vi "r4.vi"   [LabVIEW 2019]
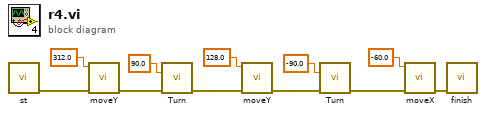
[diagram p0: block diagram]
diagram:
  n1 = call "st.vi"() -> ("Error/Flow Out"=w11:errorcluster)  [unwired: 11 in]
  n2 = call "moveY.vi"("error in (no error)"=w11, "Y"=312.0) -> ("error out"=w9:errorcluster)  [unwired: 9 in]
  n3 = call "Turn.vi"("¨¤«×"=90.0, "error in (no error)"=w9) -> ("error out"=w6:errorcluster)  [unwired: 13 in]
  n4 = call "moveY.vi"("error in (no error)"=w6, "Y"=128.0) -> ("error out"=w4:errorcluster)  [unwired: 9 in]
  n5 = call "Turn.vi"("¨¤«×"=-90.0, "error in (no error)"=w4) -> ("error out"=w3:errorcluster)  [unwired: 13 in]
  n6 = call "moveX.vi"("error in (no error)"=w3, "X"=-60.0) -> ("error out"=w1:errorcluster)  [unwired: 9 in]
  n7 = call "finish.vi"("Error/Flow In"=w1) -> ()  [unwired: 11 in]
